vi "FTW-dotNET-SQL-OpenConnectionWithEvents.vi"(5 "Connection String":string, 11 "error in":errorcluster) -> (4 "DB Connection":refnum<k24>, 6 "SQL DB Events":refnum<event-registration>, 8 "ServerVersion":string, 15 "error out":errorcluster)   [LabVIEW 2015]
uses:
  System.Data
panel:
  # "Inputs"
  # "Outputs"
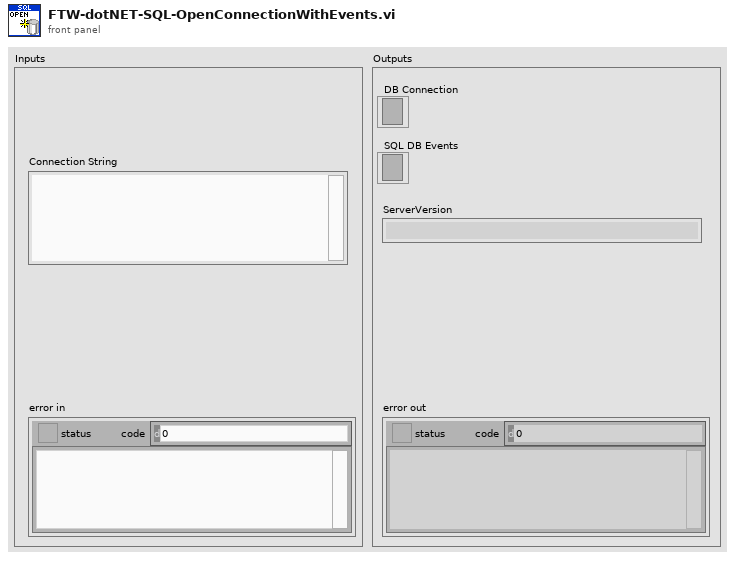
[diagram p1: front panel]
types:
  T1 = cluster{"Code":i32, "SeverityLevel":i32, "LineNumber":i32, "State":i32, "Procedure":string, "Message":string, "Source":string, "Server":string}
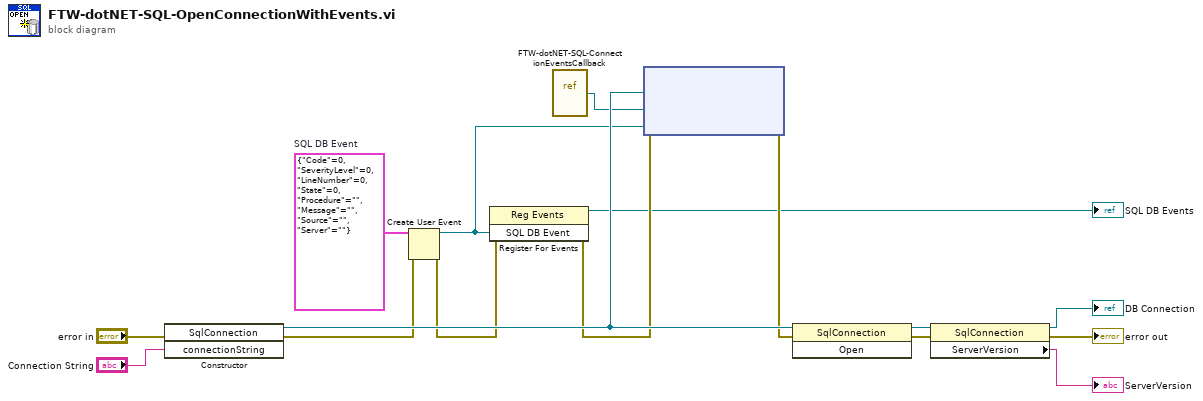
[diagram p0: block diagram]
diagram:
  w6 = T1 {"Code"=0, "SeverityLevel"=0, "LineNumber"=0, "State"=0, "Procedure"="", "Message"="", "Source"="", "Server"=""}  # SQL DB Event
  n1 = constructor class="SqlConnection"(error in="error in", "connectionString"="Connection String") -> (reference out=w9:refnum<k24>, error out=w3:errorcluster)  [unwired: 2 in, 2 out]
  n2 = Create User Event(user event datatype=w6, error in=w3) -> (user event=w2:refnum<user-event>, error out=w5:errorcluster)
  n3 = register-events(error in=w5, w2) -> (reference out=→"SQL DB Events":refnum<event-registration>, error out=w4:errorcluster)  [unwired: 1 in]
  n4 = vi-ref "FTW-dotNET-SQL-ConnectionEventsCallback.vi"() -> ("vi reference"=w7:refnum<vi>)
  n5 = node(w4, w9, w7, w2) -> (w8:errorcluster)  [unwired: 1 in, 1 out]
  n6 = invoke class="SqlConnection" method="Open"(reference=w9, error in=w8) -> (reference out=w16:refnum<k24>, error out=w15:errorcluster)  [unwired: 1 in, 1 out]
  n7 = property class="SqlConnection"(reference=w16, error in=w15) -> (reference out=→"DB Connection":refnum<k24>, error out=→"error out":errorcluster, "ServerVersion"=→"ServerVersion":string)
